vi "OE1022D_Configure Sine Out.vi"(7 "OE1022D_Configure Sine Out":T1={"Start Value(V)"=1.0, "Sine Output Amplitude (V)"=1.0, "Stop Valve(V)"=5.0, "Sine Step Valve(V)"=1.0, "Step Time(ms) "=1000, "Sine Step Percent(%)"=10.0, "SineOut Mode"=0, "Sine Run Mode"=0, "Channel"=1, "Sine Output DC (V)"=1.0} {"Sine Output DC (V)" min=-10.0 max=10.0 format="%#.3f"; "Channel" items=["A"=1, "B"=2]; "Sine Run Mode" items=["Stop", "Single", "Loop"]; "SineOut Mode" items=["Fixed", "Linear", "Log", "DC"]; "Sine Step Percent(%)" min=0.0 max=100.0 format="%#.3g"; "Step Time(ms)" min=1 max=100000; "Sine Step Valve(V)" min=0.001 max=5.0 format="%#.3g"; "Stop Valve(V)" min=0.001 max=5.0 format="%#.3g"; "Sine Output Amplitude (V)" min=0.001 max=5.0 format="%#.3g"; "Start Value(V)" min=0.001 max=5.0 format="%#.3g"}, 8 "Error in (no error)":errorcluster caption="error out（no error）", 9 "Remote Mode":u16(ring) items=["USB", "RS232", "GPIB"], 11 "VISA resource name":refnum<visa-resource-name>) -> (0 "Error out":errorcluster caption="error out", 1 "Output String":string, 3 "VISA resource  out":refnum<visa-resource-name>)   [LabVIEW 2011]
panel:
  out "SineOut Mode":u8
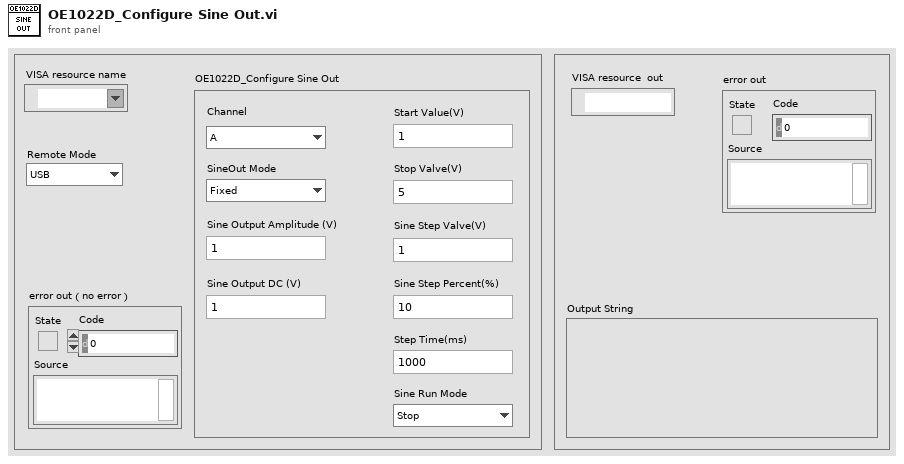
[diagram p1: front panel]
types:
  T1 = cluster{"Start Value(V)":dbl, "Sine Output Amplitude (V)":dbl, "Stop Valve(V)":dbl, "Sine Step Valve(V)":dbl, "Step Time(ms) ":u32, "Sine Step Percent(%)":dbl, "SineOut Mode":u8, "Sine Run Mode":u8, "Channel":u16, "Sine Output DC (V)":dbl}
  T2 = enum16{"ISRC", "IGND", "ICPL", "ILIN", "PHAS", "FMOD", "RSLP", "FREQ", "SWPT", "SLLM", "SULM", "SSLL", "SSLG", "STLM", "SWRM", "IRNG", "SENS", "RMOD", "OFLT", "OFSL", "SYNC", "DMOD", "HARM", "DARB", "SWVT", "SLVL", "SVLL", "SVUL", "SVSL", "SVSG", "SVTM", "SVRM", "RALL", "SNAP", "OUTP", "OAUX", "COUT", "CAUX", "COFP", "CEXP", "FPOP", "OEXP", "*IDN", "*RST", "OVLD", "INOV", "GNOV", "*PLL", "SSET", "RSET", "AGAN", "APHS", "ARSV", "ASCL", "EQCD", "EQCS", "SPED", "SRAT", "SLEN", "SSLE", "STRG", "SPRM", "STRD", "PAUS", "REST", "SPTS", "TRCA", "TEMP", "RSTU", "IHNZ", "DEQU", "SADD", "ARNG", "CSPE", "ISRCD", "IGNDD", "ICPLD", "ILIND", "PHASD", "FMODD", "RSLPD", "FREQD", "SWPTD", "SLLMD", "SULMD", "SSLLD", "SSLGD", "STLMD", "SWRMD", "SENSD", "RMODD", "OFLTD", "OFSLD", "SYNCD", "HARMD", "EQCDD", "EQCSD", "SNAPD", "OUTPD", "SWVTD", "SLVLD", "SVLLD", "SVULD", "SVSLD", "SVSGD", "SVTMD", "SVRMD", "SVDCD", "ARSVD", "AGAND", "APHSD", "ASCLD", "FPOPD", "CAUXD", "OEXPD", "SPEDD", "SRATD", "SLEND", "SSLED", "STRGD", "SPRMD", "STRDD", "PAUSD", "RESTD", "SPTSD", "TRCAD", "*IDND", "*RSTD", "INOVD", "GNOVD", "*PLLD", "SSETD", "RSETD"}
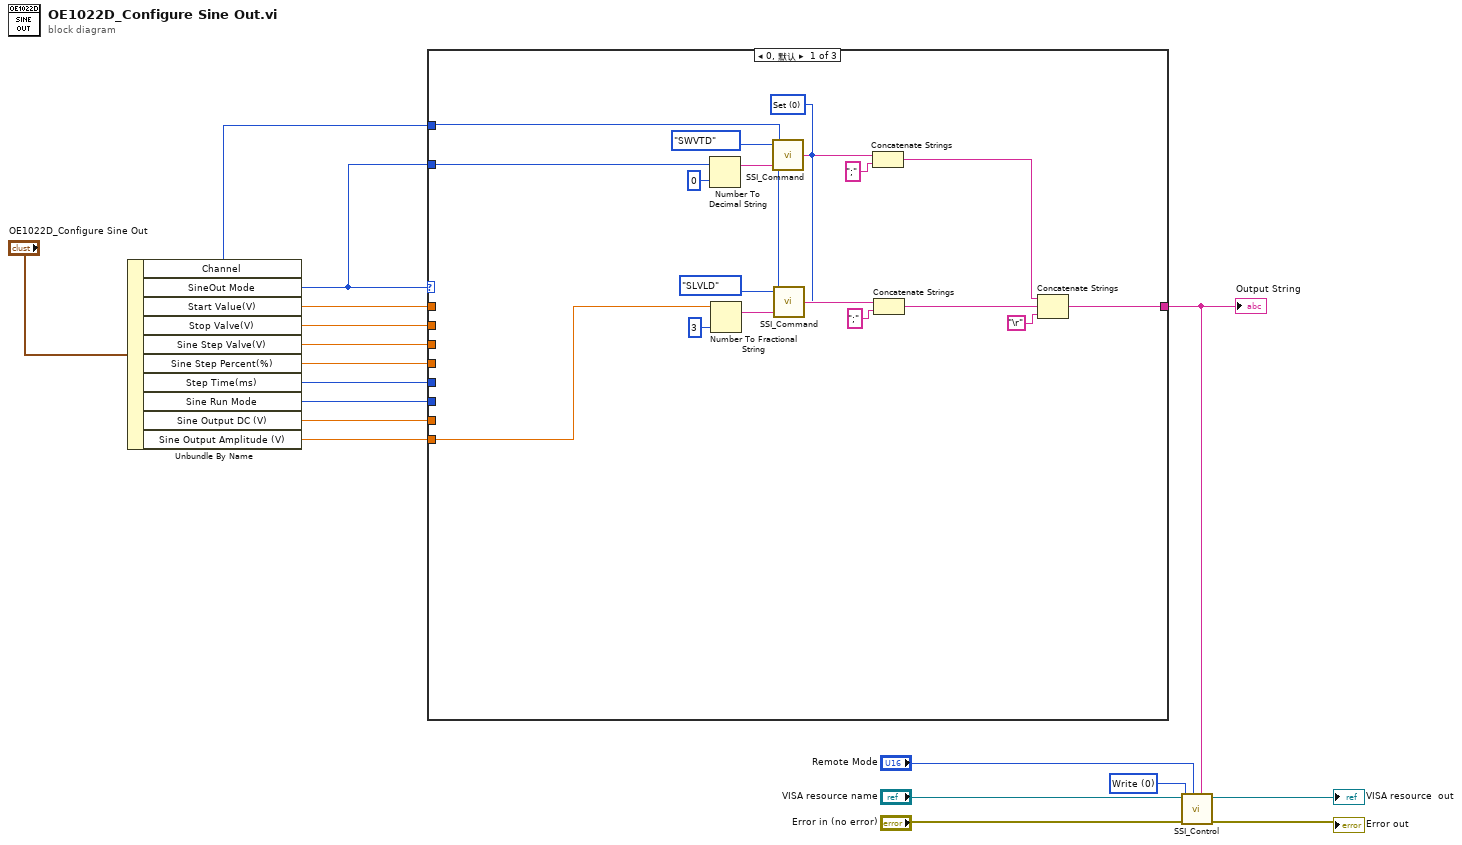
[diagram p0: block diagram]
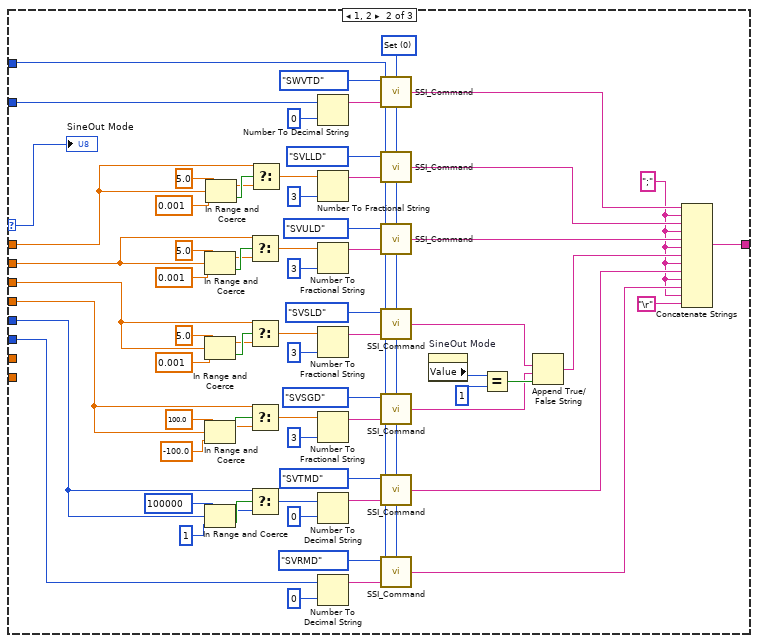
[diagram p2: hidden frame]
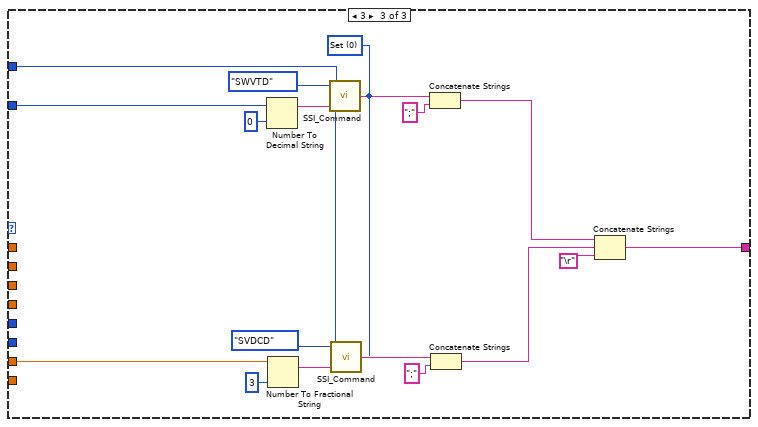
[diagram p3: hidden frame]
diagram:
  w17 = u16 0 items=["Write", "Read"] ("Control")
  n1 = Unbundle By Name("OE1022D_Configure Sine Out") -> ("Channel"=w4:u16, "SineOut Mode"=w3:u8, "Start Value(V)"=w11:dbl, "Stop Valve(V)"=w10:dbl, "Sine Step Valve(V)"=w9:dbl, "Sine Step Percent(%)"=w8:dbl, "Step Time(ms)"=w7:u32, "Sine Run Mode"=w6:u8, "Sine Output DC (V)"=w2:dbl, "Sine Output Amplitude (V)"=w1:dbl)
  n2 = case shown="0, 默认" w3 {
    selector: w3 -> [_ w38 _]
    tunnel: [w21 w62 w108] -> w5
    tunnel: w11 -> [_ w42 _]
    tunnel: w3 -> [w27 w79 w110]
    tunnel: w10 -> [_ w43 _]
    tunnel: w9 -> [_ w55 _]
    tunnel: w8 -> [_ w72 _]
    tunnel: w7 -> [_ w71 _]
    tunnel: w6 -> [_ w39 _]
    tunnel: w4 -> [w20 w40 w109]
    tunnel: w2 -> [_ _ w107]
    tunnel: w1 -> [w19 _ _]
    frame 0, Default {
      w28 = u16 0 items=["Set", "Query"] ("Opera")
      n3 = Number To Decimal String(number=w27, width (-)=i16 0 ("宽度(-)")) -> (decimal integer string=w30:string)
      n4 = Number To Fractional String(number=w19, precision (6)=i16 3 ("宽度(-)")) -> (F-format string=w34:string)  [unwired: 2 in]
      n5 = call "SSI_Command.vi"("Opera"=w28, "Paramter"=w30, "channel"=w20, "Command Type"=T2."SWVTD") -> ("Output string"=w29:string)
      n6 = call "SSI_Command.vi"("Opera"=w28, "Paramter"=w34, "channel"=w20, "Command Type"=T2."SLVLD") -> ("Output string"=w33:string)
      n7 = Concatenate Strings(w29, ";" ("替换字符串(\"\")")) -> (w22:string)
      n8 = Concatenate Strings(w33, ";" ("替换字符串(\"\")")) -> (w24:string)
      n9 = Concatenate Strings(w22, w24, "\r") -> (w21:string)
    }
    frame 1, 2 {
      w60 = ";"
      w75 = u16 0 items=["Set", "Query"] ("Opera")
      n10 = In Range and Coerce(upper limit=5.0 ("上限"), x=w43, lower limit=0.001 ("下限")) -> (coerced(x)=w53:dbl, In Range?=w54:bool)
      n11 = In Range and Coerce(upper limit=5.0 ("上限"), x=w55, lower limit=0.001 ("下限")) -> (coerced(x)=w58:dbl, In Range?=w59:bool)
      n12 = In Range and Coerce(upper limit=100.0 ("上限"), x=w72, lower limit=-100.0 ("下限")) -> (coerced(x)=w82:dbl, In Range?=w83:bool)
      n13 = In Range and Coerce(upper limit=u32 100000 ("上限"), x=w71, lower limit=u32 1 ("下限")) -> (coerced(x)=w86:u32, In Range?=w87:bool)
      n14 = In Range and Coerce(upper limit=5.0 ("上限"), x=w42, lower limit=0.001 ("下限")) -> (coerced(x)=w47:dbl, In Range?=w48:bool)
      n15 = Select(t=w43, s=w54, f=w53) -> (s? t:f=w50:dbl)
      n16 = Select(t=w55, s=w59, f=w58) -> (s? t:f=w49:dbl)
      n17 = Select(t=w72, s=w83, f=w82) -> (s? t:f=w73:dbl)
      n18 = Select(t=w71, s=w87, f=w86) -> (s? t:f=w74:u32)
      n19 = Select(t=w42, s=w48, f=w47) -> (s? t:f=w44:dbl)
      n20 = Number To Decimal String(number=w79, width (-)=i16 0 ("精度(6)")) -> (decimal integer string=w101:string)
      n21 = Number To Fractional String(number=w44, precision (6)=i16 3 ("精度(6)")) -> (F-format string=w98:string)  [unwired: 2 in]
      n22 = Number To Fractional String(number=w50, precision (6)=i16 3 ("精度(6)")) -> (F-format string=w95:string)  [unwired: 2 in]
      n23 = Number To Fractional String(number=w49, precision (6)=i16 3 ("精度(6)")) -> (F-format string=w92:string)  [unwired: 2 in]
      n24 = Number To Fractional String(number=w73, precision (6)=i16 3 ("精度(6)")) -> (F-format string=w89:string)  [unwired: 2 in]
      n25 = Number To Decimal String(number=w74, width (-)=i16 0 ("精度(6)")) -> (decimal integer string=w104:string)
      n26 = Number To Decimal String(number=w39, width (-)=i16 0 ("精度(6)")) -> (decimal integer string=w77:string)
      n27 = call "SSI_Command.vi"("Opera"=w75, "Paramter"=w101, "channel"=w40, "Command Type"=T2."SWVTD") -> ("Output string"=w68:string)
      n28 = call "SSI_Command.vi"("Opera"=w75, "Paramter"=w98, "channel"=w40, "Command Type"=T2."SVLLD") -> ("Output string"=w67:string)
      n29 = call "SSI_Command.vi"("Opera"=w75, "Paramter"=w95, "channel"=w40, "Command Type"=T2."SVULD") -> ("Output string"=w66:string)
      n30 = call "SSI_Command.vi"("Opera"=w75, "Paramter"=w92, "channel"=w40, "Command Type"=T2."SVSLD") -> ("Output string"=w69:string)
      n31 = call "SSI_Command.vi"("Opera"=w75, "Paramter"=w89, "channel"=w40, "Command Type"=T2."SVSGD") -> ("Output string"=w70:string)
      n32 = call "SSI_Command.vi"("Opera"=w75, "Paramter"=w104, "channel"=w40, "Command Type"=T2."SVTMD") -> ("Output string"=w64:string)
      n33 = call "SSI_Command.vi"("Opera"=w75, "Paramter"=w77, "channel"=w40, "Command Type"=T2."SVRMD") -> ("Output string"=w63:string)
      n34 = property on="SineOut Mode" class="DigNum (严格)"() -> ("Value"=w37:u8)  [unwired: 2 in, 2 out]
      n35 = Equal?(x=w37, y=u8 1 ("x")) -> (x = y?=w106:bool)
      n36 = Append True/False String(1:w106, 2:w70, 3:w69) -> (0:w65:string)  [unwired: 1 in]
      n37 = Concatenate Strings(w68, w60, w67, w60, w66, w60, w65, w60, w64, w60, w63, w60, "\r") -> (w62:string)
      "SineOut Mode" <- w38
    }
    frame 3 {
      w116 = u16 0 items=["Set", "Query"] ("Opera")
      n38 = Number To Decimal String(number=w110, width (-)=i16 0 ("宽度(-)")) -> (decimal integer string=w118:string)
      n39 = Number To Fractional String(number=w107, precision (6)=i16 3 ("宽度(-)")) -> (F-format string=w122:string)  [unwired: 2 in]
      n40 = call "SSI_Command.vi"("Opera"=w116, "Paramter"=w118, "channel"=w109, "Command Type"=T2."SWVTD") -> ("Output string"=w117:string)
      n41 = call "SSI_Command.vi"("Opera"=w116, "Paramter"=w122, "channel"=w109, "Command Type"=T2."SVDCD") -> ("Output string"=w121:string)
      n42 = Concatenate Strings(w117, ";" ("替换字符串(\"\")")) -> (w111:string)
      n43 = Concatenate Strings(w121, ";" ("替换字符串(\"\")")) -> (w113:string)
      n44 = Concatenate Strings(w111, w113, "\r") -> (w108:string)
    }
  }
  "Output String" <- w5
  n45 = call "SSI_Control.vi"("Write Buffer"=w5, "Remote Mode"="Remote Mode", "Error in (no error)"="Error in (no error)", "Control"=w17, "VISA resource name"="VISA resource name") -> ("Error out"=→"Error out":errorcluster, "VISA resource  out"=→"VISA resource  out":refnum<visa-resource-name>)  [unwired: 3 in, 2 out]
